vi "Preview Waveform.vi"(4 "Decimation Multiple":u16, 6 "Max Size":i64, 8 "Channel #":i8, 9 "In Use?":bool, 10 "New Y Values":dbl[][](array[numeric]), 11 "Old Y Values":dbl[][](array[numeric])) -> (3 "Output Y Values":dbl[](array[numeric]))   [LabVIEW 2014]
panel:
  # "Preview Waveform"
  # "Inputs"
  # "Outputs"
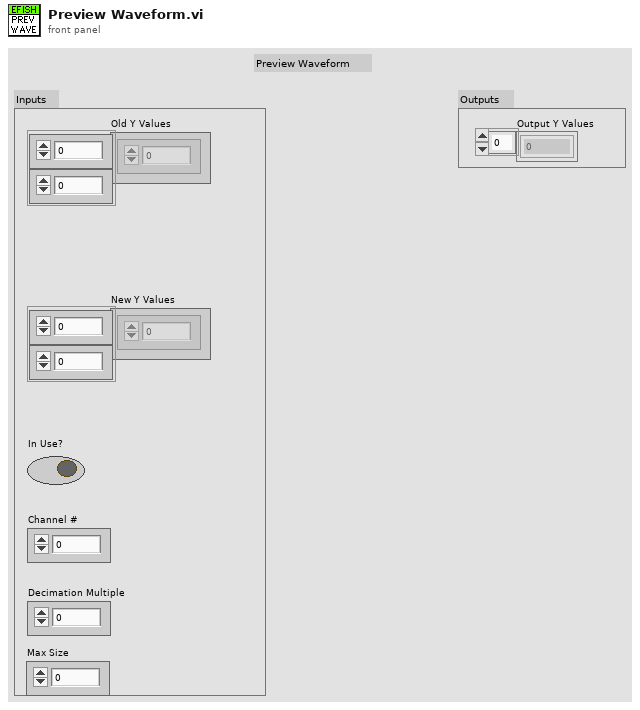
[diagram p1: front panel]
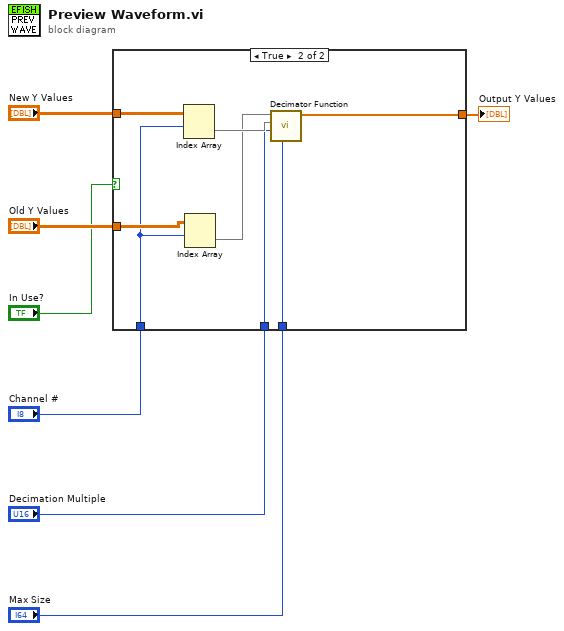
[diagram p0: block diagram]
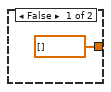
[diagram p2: hidden frame]
diagram:
  n1 = case shown="True" "In Use?" {
    tunnel: "New Y Values" -> [_ w16]
    tunnel: "Old Y Values" -> [_ w14]
    tunnel: "Channel #" -> [_ w13]
    tunnel: "Decimation Multiple" -> [_ w11]
    tunnel: [dbl[] [] ("Output Y Values") w10] -> w2
    tunnel: "Max Size" -> [_ w9]
    frame False {
    }
    frame True {
      n2 = Index Array(array=w16, index (row)=w13) -> (element=w15:dbl[])  [unwired: 1 in]
      n3 = Index Array(array=w14, index (row)=w13) -> (element=w12:dbl[])  [unwired: 1 in]
      n4 = call "Decimator Function.vi"("Max Size (10K)"=w9, "Decimation #"=w11, "Input Y values New"=w15, "Input Y values Old"=w12) -> ("Output Y Values"=w10:dbl[])  [unwired: 7 in]
    }
  }
  "Output Y Values" <- w2
